vi "Source.Write.Range.Base10 (U64).vi"(5 "<= max? (T)":bool=TRUE, 7 ">= min? (T)":bool=TRUE, 8 "min":u64 format="%d bytes", 9 "max":u64 format="%d bytes", 10 "value":u64 format="%d bytes", 11 "error in":errorcluster) -> (3 "error out":errorcluster)   [LabVIEW 2016, in "Memory Manager.lvlib" / "Static Error Handling.lvlib"]
uses:
  Static Error Handling.lvlib
panel:
  out "new offset":i32
  in  "offset":i32
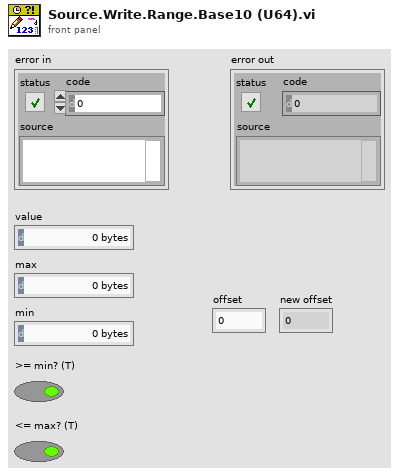
[diagram p1: front panel]
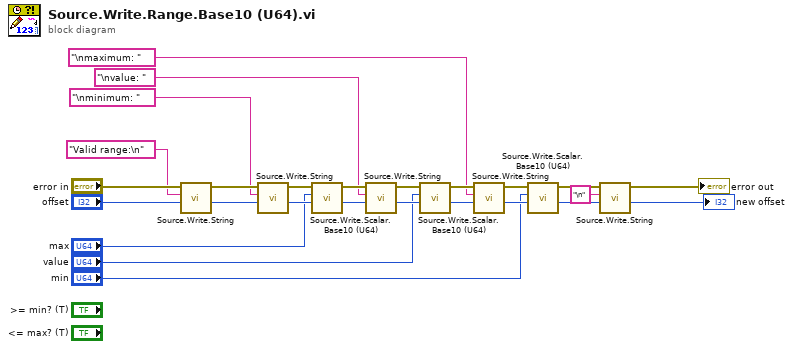
[diagram p0: block diagram]
diagram:
  n1 = call "Source.Write.String.vi"("offset"="offset", "string"="Valid range:\n", "error in"="error in") -> ("new offset"=w5:i32, "error out"=w6:errorcluster)  [unwired: 7 in]
  n2 = call "Source.Write.String.vi"("offset"=w5, "string"="\nminimum: ", "error in"=w6) -> ("new offset"=w23:i32, "error out"=w26:errorcluster)  [unwired: 7 in]
  n3 = call "Source.Write.Scalar.Base10 (U64).vi"("offset"=w23, "value"="max", "error in"=w26) -> ("new offset"=w24:i32, "error out"=w25:errorcluster)  [unwired: 7 in]
  n4 = call "Source.Write.String.vi"("offset"=w24, "string"="\nvalue: ", "error in"=w25) -> ("new offset"=w20:i32, "error out"=w21:errorcluster)  [unwired: 7 in]
  n5 = call "Source.Write.Scalar.Base10 (U64).vi"("offset"=w20, "value"="value", "error in"=w21) -> ("new offset"=w18:i32, "error out"=w19:errorcluster)  [unwired: 7 in]
  n6 = call "Source.Write.String.vi"("offset"=w18, "string"="\nmaximum: ", "error in"=w19) -> ("new offset"=w16:i32, "error out"=w17:errorcluster)  [unwired: 7 in]
  n7 = call "Source.Write.Scalar.Base10 (U64).vi"("offset"=w16, "value"="min", "error in"=w17) -> ("new offset"=w12:i32, "error out"=w14:errorcluster)  [unwired: 7 in]
  n8 = call "Source.Write.String.vi"("offset"=w12, "string"="\n", "error in"=w14) -> ("new offset"=→"new offset":i32, "error out"=→"error out":errorcluster)  [unwired: 7 in]
